vi "initGyro.vi"   [LabVIEW 2016]
uses:
  #defines.ctl
  GLOBALS.vi
types:
  T1 = typedef "#defines.ctl" = i16
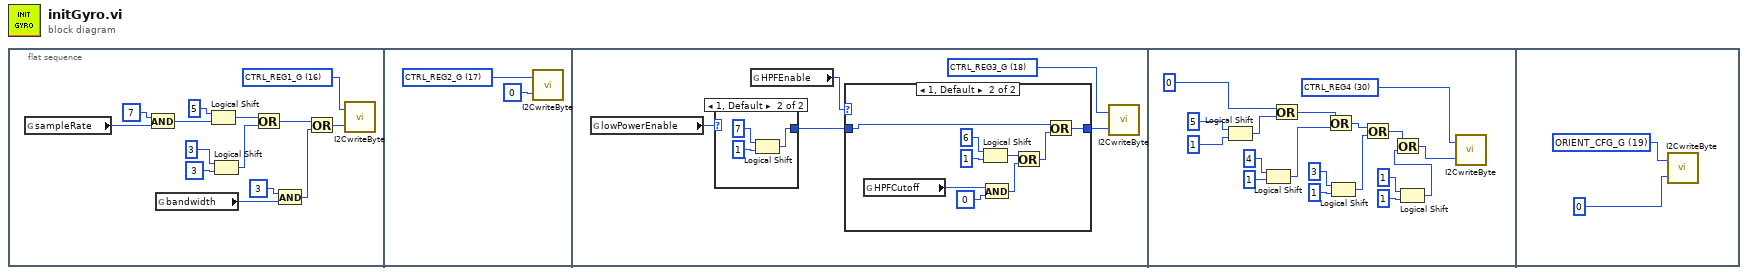
[diagram p0: block diagram]
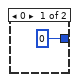
[diagram p3: hidden frame]
diagram:
  n1 = flat-sequence {
    frame #0 {
      w2 = T1 16 items=["CTRL_REG9_G"=35, "STATUS_REG_1"=39, "OUT_X_L_XL"=40, "FIFO_CTRL"=46, "FIFO_SRC"=47, "CTRL_REG4_G"=30, "OUT_X_L_G"=24, "OUT_TEMP_L"=21, "INT_GEN_SRC_G"=20, "ORIENT_CFG_G"=19, "CTRL_REG3_G"=18, "CTRL_REG2_G"=17, "CTRL_REG1_G"=16, "WHO_AM_I_XG"=15] ("Ring")
      n2 = global read "GLOBALS.vi" "sampleRate"() -> (w14:u8)
      n3 = And(x=u8 7, y=w14) -> (x .and. y?=w11:u8)
      n4 = global read "GLOBALS.vi" "bandwidth"() -> (w4:u8)
      n5 = Logical Shift(y=5, x=w11) -> (x << y=w10:u8)
      n6 = Logical Shift(y=3, x=u8 3) -> (x << y=w7:u8)
      n7 = Or(x=w10, y=w7) -> (x .or. y?=w6:u8)
      n8 = And(x=u8 3, y=w4) -> (x .and. y?=w3:u8)
      n9 = Or(x=w6, y=w3) -> (x .or. y?=w1:u8)
      n10 = call "I2CwriteByte.vi"("data"=w1, "subAddress"=w2) -> ()  [unwired: 1 in]
    }
    frame #1 {
      w16 = T1 17 items=["CTRL_REG9_G"=35, "STATUS_REG_1"=39, "OUT_X_L_XL"=40, "FIFO_CTRL"=46, "FIFO_SRC"=47, "CTRL_REG4_G"=30, "OUT_X_L_G"=24, "OUT_TEMP_L"=21, "INT_GEN_SRC_G"=20, "ORIENT_CFG_G"=19, "CTRL_REG3_G"=18, "CTRL_REG2_G"=17, "CTRL_REG1_G"=16, "WHO_AM_I_XG"=15] ("Ring")
      n11 = call "I2CwriteByte.vi"("data"=u8 0, "subAddress"=w16) -> ()  [unwired: 1 in]
    }
    frame #2 {
      w17 = T1 18 items=["CTRL_REG9_G"=35, "STATUS_REG_1"=39, "OUT_X_L_XL"=40, "FIFO_CTRL"=46, "FIFO_SRC"=47, "CTRL_REG4_G"=30, "OUT_X_L_G"=24, "OUT_TEMP_L"=21, "INT_GEN_SRC_G"=20, "ORIENT_CFG_G"=19, "CTRL_REG3_G"=18, "CTRL_REG2_G"=17, "CTRL_REG1_G"=16, "WHO_AM_I_XG"=15] ("Ring")
      n12 = global read "GLOBALS.vi" "lowPowerEnable"() -> (w21:u8)
      n13 = case shown="1, Default" w21 {
        tunnel: [0 w33] -> w19
        frame 0 {
        }
        frame 1, Default {
          n14 = Logical Shift(y=7, x=1) -> (x << y=w33:i32)
        }
      }
      n15 = global read "GLOBALS.vi" "HPFEnable"() -> (w20:u8)
      n16 = case shown="1, Default" w20 {
        tunnel: [w22 w23] -> w18
        tunnel: w19 -> [w22 w29]
        frame 0 {
        }
        frame 1, Default {
          n17 = global read "GLOBALS.vi" "HPFCutoff"() -> (w28:u8)
          n18 = Logical Shift(y=6, x=1) -> (x << y=w26:i32)
          n19 = And(x=w28, y=u8 0) -> (x .and. y?=w25:u8)
          n20 = Or(x=w26, y=w25) -> (x .or. y?=w24:i32)
          n21 = Or(x=w29, y=w24) -> (x .or. y?=w23:i32)
        }
      }
      n22 = call "I2CwriteByte.vi"("data"=w18, "subAddress"=w17) -> ()  [unwired: 1 in]
    }
    frame #3 {
      w36 = T1 30 items=["CTRL_REG9"=35, "STATUS_REG_1"=39, "OUT_X_L_XL"=40, "FIFO_CTRL"=46, "FIFO_SRC"=47, "CTRL_REG4"=30, "OUT_X_L_G"=24, "OUT_TEMP_L"=21, "INT_GEN_SRC_G"=20, "ORIENT_CFG_G"=19, "CTRL_REG3_G"=18, "CTRL_REG2_G"=17, "CTRL_REG1_G"=16, "WHO_AM_I_XG"=15] ("Ring")
      n23 = Logical Shift(y=5, x=1) -> (x << y=w44:i32)
      n24 = Logical Shift(y=4, x=1) -> (x << y=w42:i32)
      n25 = Or(x=0, y=w44) -> (x .or. y?=w43:i32)
      n26 = Or(x=w43, y=w42) -> (x .or. y?=w41:i32)
      n27 = Logical Shift(y=3, x=1) -> (x << y=w40:i32)
      n28 = Or(x=w41, y=w40) -> (x .or. y?=w39:i32)
      n29 = Logical Shift(y=1, x=1) -> (x << y=w38:i32)
      n30 = Or(x=w39, y=w38) -> (x .or. y?=w37:i32)
      n31 = call "I2CwriteByte.vi"("data"=w37, "subAddress"=w36) -> ()  [unwired: 1 in]
    }
    frame #4 {
      w54 = T1 19 items=["CTRL_REG9"=35, "STATUS_REG_1"=39, "OUT_X_L_XL"=40, "FIFO_CTRL"=46, "FIFO_SRC"=47, "CTRL_REG4"=30, "OUT_X_L_G"=24, "OUT_TEMP_L"=21, "INT_GEN_SRC_G"=20, "ORIENT_CFG_G"=19, "CTRL_REG3_G"=18, "CTRL_REG2_G"=17, "CTRL_REG1_G"=16, "WHO_AM_I_XG"=15] ("Ring")
      n32 = call "I2CwriteByte.vi"("data"=0, "subAddress"=w54) -> ()  [unwired: 1 in]
    }
  }
